vi "Simulate RTD PointByPoint.vi"() -> ()   [LabVIEW 8.6]
uses:
  vi.lib/UeiDaq/UeiDaqConfigureTimingForSimpleIO.vi
  vi.lib/UeiDaq/UeiDaqWriteOneScaledScan.vi
panel:
  in  "Short Max Duration (us)":u32
  in  "Shorted channel mask":bool[](array[boolean])
  in  "RTD Settings":T1 {"Temperature Scale" items=["Celsius", "Fahrenheit", "Kelvin", "Rankine"]; "RTD type" items=["3750", "3850", "3902", "3911", "3916", "3920", "3926", "3928", "Custom"]}
  in  "Open channel mask":bool[](array[boolean])
  in  "Output Values":dbl[](array[numeric])
  in  "AO Resource":string
  in  "Refresh rate (ms)":u32
  in  "stop":bool
  # "Simulate RTD on RTD-388"
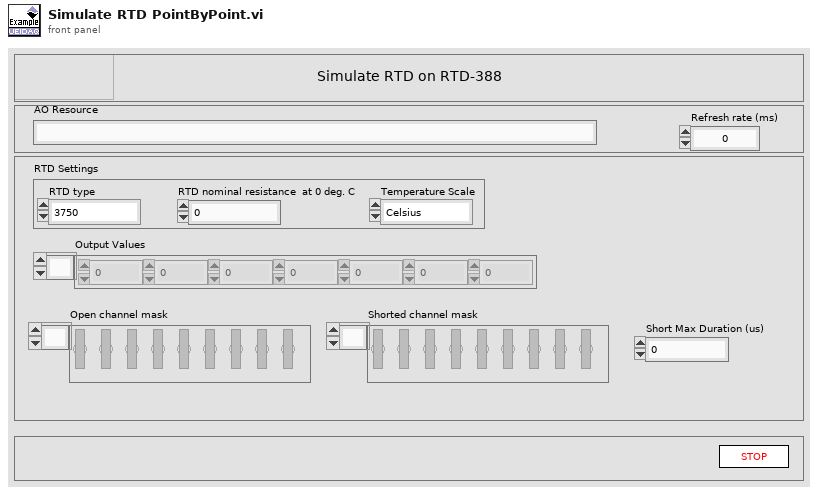
[diagram p1: front panel]
types:
  T1 = cluster{"RTD type":u16, "RTD nominal resistance  at 0 deg. C":dbl, "Temperature Scale":i32}
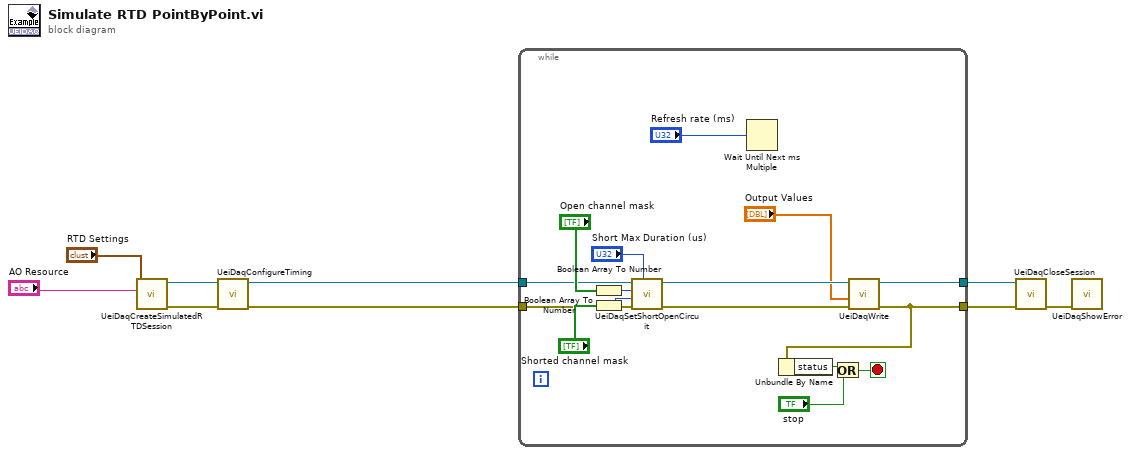
[diagram p0: block diagram]
diagram:
  n1 = call "UeiDaqCreateSimulatedRTDSession.vi"("RTD Settings"="RTD Settings", "Resource"="AO Resource") -> ("error out"=w8:errorcluster, "UeiDaq Refnum Out"=w9:refnum<k20>)  [unwired: 8 in]
  n2 = call-poly "UeiDaqConfigureTiming.vi"("error in (no error)"=w8, "UeiDaq Refnum In"=w9) -> ("error out"=w4:errorcluster, "UeiDaq Refnum Out"=w7:refnum<k20>)  [unwired: 8 out]
  n3 = while {
    tunnel: w7 -> [w15]
    tunnel: [w21] -> w5
    tunnel: w4 -> [w14]
    tunnel: [w11] -> w1
    stop <- w24 stop-if-true
    n4 = Boolean Array To Number(Boolean array="Open channel mask") -> (number=w19:u32)
    n5 = Boolean Array To Number(Boolean array="Shorted channel mask") -> (number=w17:u32)
    n6 = call "UeiDaqSetShortOpenCircuit.vi"("UeiDaq Refnum In"=w15, "Open Mask"=w19, "Short Mask"=w17, "error in (no error)"=w14, "Short Max Duration (us)"="Short Max Duration (us)") -> ("UeiDaq Refnum Out"=w12:refnum<k20>, "error out"=w13:errorcluster)  [unwired: 4 in]
    n7 = Wait Until Next ms Multiple(millisecond multiple="Refresh rate (ms)") -> ()  [unwired: 1 out]
    n8 = call-poly "UeiDaqWrite.vi"("error in (no error)"=w13, "Scaled Data"="Output Values", "UeiDaq Refnum In"=w12) -> ("error out"=w21:errorcluster, "UeiDaq Refnum Out"=w11:refnum<k20>)  [unwired: 1 in, 6 out]
    n9 = Unbundle By Name(w21) -> ("status"=w22:bool)
    n10 = Or(x=w22, y="stop") -> (x .or. y?=w24:bool)
  }
  n11 = call "UeiDaqCloseSession.vi"("error in (no error)"=w5, "UeiDaq Refnum In"=w1) -> ("error out"=w3:errorcluster)  [unwired: 1 in, 8 out]
  n12 = call "UeiDaqShowError.vi"("error in (no error)"=w3) -> ()  [unwired: 2 in, 9 out]
